vi "Chroma 1905x Series Delay.vi"(8 "error in (no error)":errorcluster, 10 "Time Delay ms":u32, 11 "VISA resource name":refnum<visa-resource-name>) -> (0 "error out":errorcluster, 3 "VISA resource name 2":refnum<visa-resource-name>)   [LabVIEW 2025]
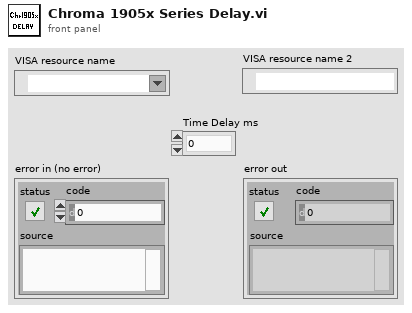
[diagram p1: front panel]
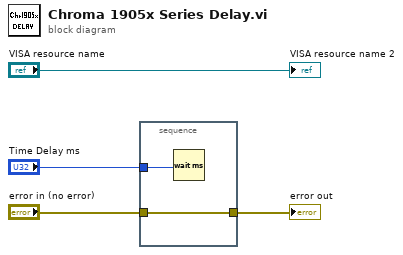
[diagram p0: block diagram]
diagram:
  n1 = stacked-sequence {
    tunnel: "error in (no error)" -> [w6]
    tunnel: [w6] -> w3
    tunnel: "Time Delay ms" -> [w5]
    frame #0 {
      n2 = Wait (ms)(milliseconds to wait=w5) -> ()  [unwired: 1 out]
    }
  }
  "error out" <- w3
  "VISA resource name 2" <- "VISA resource name"
